vi "Drive Check for New Command.vi"(9 "input cluster":T6, 10 "Wait time (ms)":dbl, 11 "Finished?":bool) -> (0 "Completion":T4, 1 "Subsystem Name":string, 2 "Current Command":T1, 3 "Initial Trace String":string, 4 "Next Command":T6)   [LabVIEW 2017]
doc: "This VI is called for each controller loop iteration. It checks for new commands, updates timing data, and upon completion, notifies and waiting commands."
uses:
  Drive Setpoints.ctl
  Drive Operations.ctl
  <vilib>/Rock Robotics/WPI/Framework/Command Status Info.ctl
  <vilib>/Rock Robotics/WPI/Framework/Completion Status.ctl
  <vilib>/Rock Robotics/WPI/Framework/Completion Notifier.ctl
  Drive Published Globals.vi
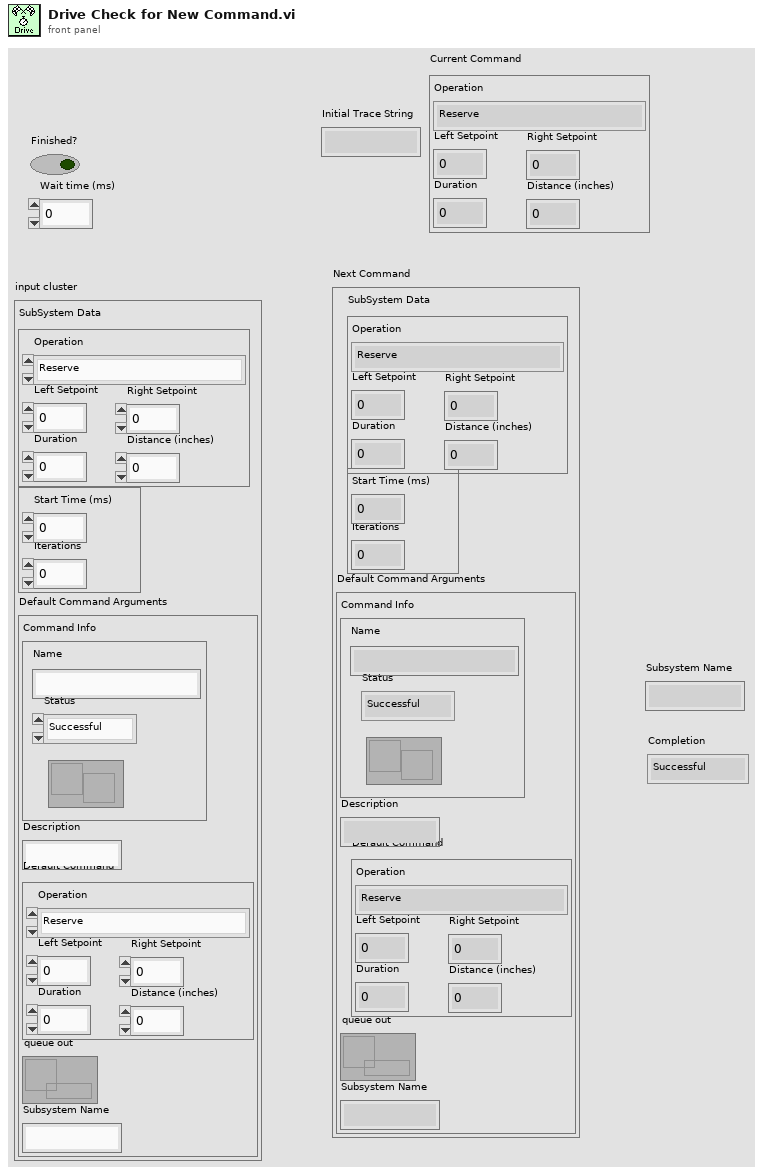
[diagram p1: front panel]
types:
  T1 = typedef "Drive Setpoints.ctl" = cluster{"Operation":T2, "Left Setpoint":dbl, "Right Setpoint":dbl, "Duration":dbl, "Distance (inches)":dbl}
  T2 = typedef "Drive Operations.ctl" = enum16{"Reserve", "Read Current", "Immediate", "Drive for Time", "Drive for Distance"}
  T3 = typedef "Command Status Info.ctl" = cluster{"Name":string, "Status":T4, "notifier out":T5}
  T4 = typedef "Completion Status.ctl" = enum16{"Successful", "Aborted", "Incomplete"}
  T5 = typedef "Completion Notifier.ctl" = refnum<notifier>
  T6 = cluster{"SubSystem Data":T1, cluster{"Start Time (ms)":u32, "Iterations":i32}, "Default Command Arguments":cluster{"Command Info":T3, "Description":string, "Default Command":T1, "queue out":refnum<queue>, "Subsystem Name":string}}
  T7 = cluster{"Command Info":T3, "Description":string, "Default Command":T1, "queue out":refnum<queue>, "Subsystem Name":string}
  T8 = cluster{"Default Command":T1, "Command Info":T3, "Description":string}
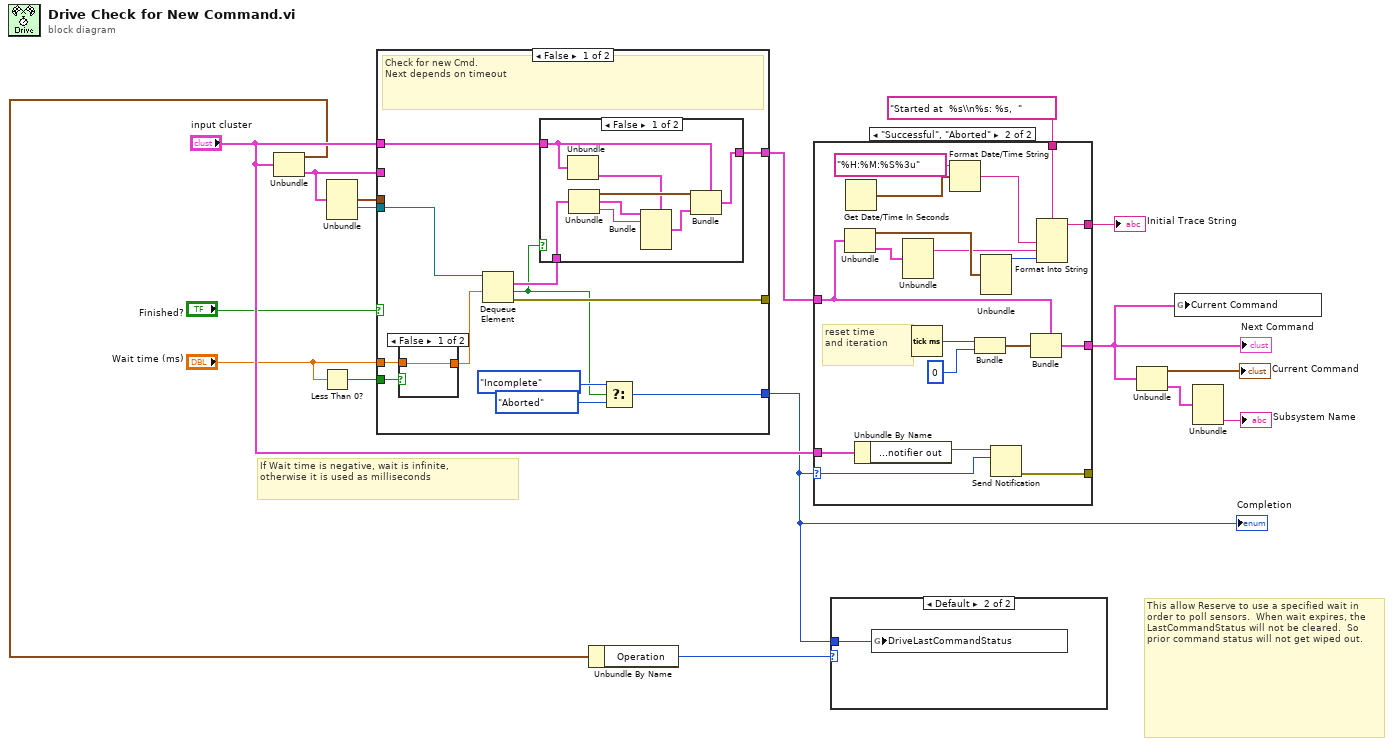
[diagram p0: block diagram]
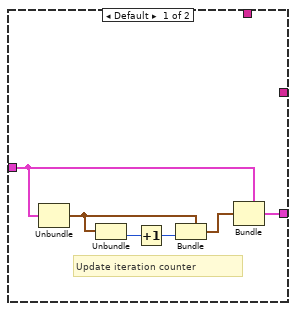
[diagram p3: hidden frame]
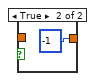
[diagram p5: hidden frame]
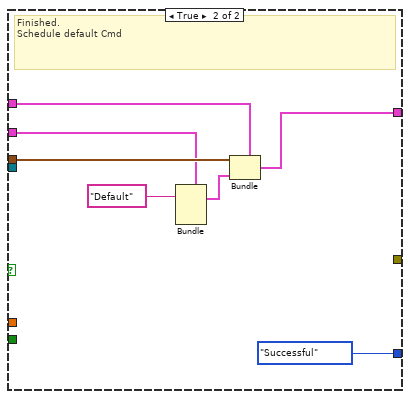
[diagram p6: hidden frame]
diagram:
  # "This allow Reserve to use a specified wait in order to poll sensors.  When wait expires, the LastCommandStatus will not be cleared.  So prior command status will not get wiped out."
  # "If Wait time is negative, wait is infinite,\notherwise it is used as milliseconds"
  n1 = Unbundle("input cluster") -> ("SubSystem Data"=w2:T1, "Default Command Arguments"=w7:T7)  [unwired: 1 out]
  n2 = Less Than 0?(x="Wait time (ms)") -> (x < 0?=w5:bool)
  n3 = Unbundle(w7) -> ("Default Command"=w10:T1, "queue out"=w11:refnum<queue>)  [unwired: 3 out]
  n4 = case shown="False" "Finished?" {
    tunnel: [w25 w46] -> w14
    tunnel: w5 -> [w19 _]
    tunnel: [w29 Completion_Status."Successful"] -> w3
    tunnel: [w22 _] -> _
    tunnel: w11 -> [w24 _]
    tunnel: "input cluster" -> [w26 w45]
    tunnel: w10 -> [_ w44]
    tunnel: w7 -> [_ w42]
    tunnel: "Wait time (ms)" -> [w18 _]
    frame False {
      # "Check for new Cmd.\nNext depends on timeout"
      n5 = case shown="False" w19 {
        tunnel: [w39 -1] -> w23
        tunnel: w18 -> [w39 _]
        frame False {
        }
        frame True {
        }
      }
      n6 = Dequeue Element(queue=w24, timeout in ms (-1)=w23) -> (element=w21:T8, timed out?=w20:bool, error out=w22:errorcluster)  [unwired: 1 in, 1 out]
      n7 = case shown="False" w20 {
        tunnel: w21 -> [w37 _]
        tunnel: w26 -> [w34 w38]
        tunnel: [w30 w38] -> w25
        frame False {
          n8 = Unbundle(w34) -> ("Default Command Arguments"=w33:T7)  [unwired: 2 out]
          n9 = Unbundle(w37) -> ("Default Command"=w36:T1, "Command Info"=w31:T3, "Description"=w32:string)
          n10 = Bundle(cluster=w33, "Command Info"=w31, "Description"=w32) -> (w35:T7)  [unwired: 3 in]
          n11 = Bundle(cluster=w34, "SubSystem Data"=w36, "Default Command Arguments"=w35) -> (w30:T6)  [unwired: 1 in]
        }
        frame True {
        }
      }
      n12 = Select(t=Completion_Status."Incomplete", s=w20, f=Completion_Status."Aborted") -> (s? t:f=w29:T4)
    }
    frame True {
      # "Finished.\nSchedule default Cmd"
      n13 = Bundle(cluster=w42, "Description"="Default") -> (w43:T7)  [unwired: 4 in]
      n14 = Bundle(cluster=w45, "SubSystem Data"=w44, "Default Command Arguments"=w43) -> (w46:T6)  [unwired: 1 in]
    }
  }
  "Completion" <- w3
  n15 = Unbundle By Name(w2) -> ("Operation"=w1:T2)
  n16 = case shown="\"Successful\", \"Aborted\"" w3 {
    selector: w3 -> [_ w71]
    tunnel: "input cluster" -> [_ w59]
    tunnel: "Started at  %s\\n%s: %s,  " ("format string") -> [_ w68]
    tunnel: [_ w67] -> w16
    tunnel: w14 -> [w50 w60]
    tunnel: [w51 w64] -> w6
    tunnel: [_ w61] -> _
    frame Default {
      # "Update iteration counter"
      n17 = Unbundle(w50) -> (w49:cluster{"Start Time (ms)":u32, "Iterations":i32})  [unwired: 2 out]
      n18 = Unbundle(w49) -> ("Iterations"=w52:i32)  [unwired: 1 out]
      n19 = Increment(x=w52) -> (x+1=w53:i32)
      n20 = Bundle(cluster=w49, "Iterations"=w53) -> (w48:cluster{"Start Time (ms)":u32, "Iterations":i32})  [unwired: 1 in]
      n21 = Bundle(cluster=w50, w48) -> (w51:T6)  [unwired: 2 in]
    }
    frame "Successful", "Aborted" {
      # "reset time\nand iteration"
      n22 = Unbundle(w60) -> ("SubSystem Data"=w66:T1, "Default Command Arguments"=w62:T7)  [unwired: 1 out]
      n23 = Get Date/Time In Seconds() -> (seconds since 1Jan1904=w55:timestamp)
      n24 = Unbundle By Name(w59) -> ("Default Command Arguments.Command Info.notifier out"=w70:T5)
      n25 = Unbundle(w62) -> ("Description"=w57:string)  [unwired: 4 out]
      n26 = Tick Count (ms)() -> (millisecond timer value=w58:u32)
      n27 = Format Date/Time String(time format string (%c)="%H:%M:%S%3u", seconds (now)=w55) -> (date/time string=w54:string)  [unwired: 1 in]
      n28 = Bundle("millisecond timer value"=w58, 0) -> (w63:cluster{"millisecond timer value":u32, i32})  [unwired: 1 in]
      n29 = Unbundle(w66) -> ("Operation"=w69:T2)  [unwired: 4 out]
      n30 = Send Notification(notification=w71, notifier=w70) -> (error out=w61:errorcluster)  [unwired: 1 in, 1 out]
      n31 = Bundle(cluster=w60, w63) -> (w64:T6)  [unwired: 2 in]
      n32 = Format Into String(format string=w68, w54, w57, w69) -> (resulting string=w67:string)  [unwired: 2 in, 1 out]
    }
  }
  "Next Command" <- w6
  "Initial Trace String" <- w16
  n33 = case shown="Default" w1 {
    tunnel: w3 -> [_ w72]
    frame "Reserve" {
      # "If interrupted by Reserve,\nDon't update LastCommandStatus"
    }
    frame Default {
      n34 = global write "Drive Published Globals.vi" "DriveLastCommandStatus"(w72) -> ()
    }
  }
  n35 = Unbundle(w6) -> ("SubSystem Data"=→"Current Command":T1, "Default Command Arguments"=w9:T7)  [unwired: 1 out]
  n36 = global write "Drive Published Globals.vi" "Current Command"(w6) -> ()
  n37 = Unbundle(w9) -> ("Subsystem Name"=→"Subsystem Name":string)  [unwired: 4 out]
